vi "Excel_Voltage.vi"(7 "duanVoltage":dbl[](array[numeric]), 8 "error in (no error)":errorcluster, 10 "Report path in":path, 11 "report in":refnum<class "NI_report.lvclass">) -> (0 "error out":errorcluster, 2 "Report path out":path, 3 "report out":refnum<class "NI_report.lvclass">)   [LabVIEW 2015]
doc: "如果duanVoltage=-1，报表中输出‘-’。"
uses:
  <vilib>/Utility/NIReport.llb/NI_report.lvclass
  <vilib>/addons/_office/NI_ReportGenerationToolkit.lvlib
panel:
  in  "start(-1,-1)":cluster{"row":i32, "column":i32}
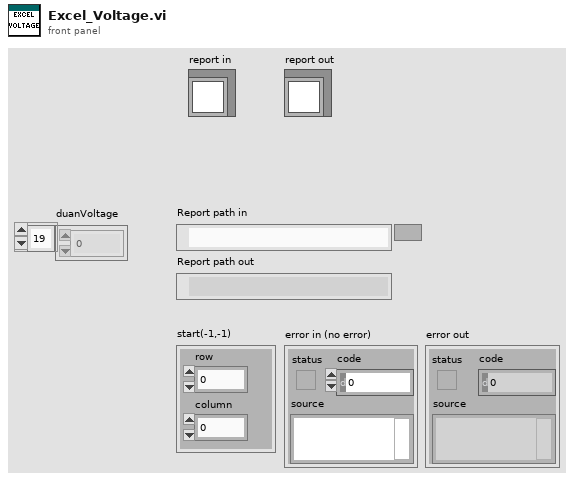
[diagram p1: front panel]
types:
  T1 = enum16{"Standard Report", "HTML", "Word", "Excel"}
  T2 = enum16{"maximized", "minimized", "normal", "no change"}
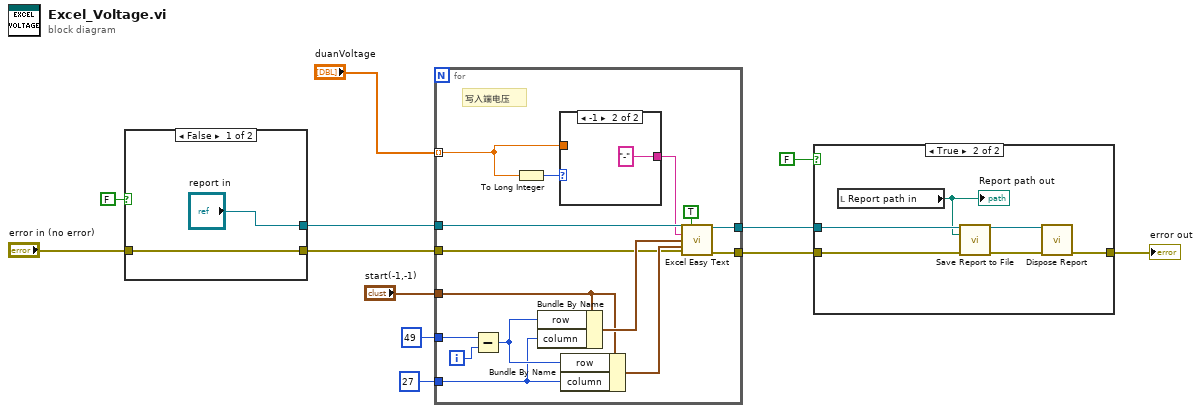
[diagram p0: block diagram]
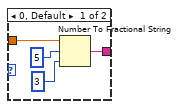
[diagram p2: hidden frame]
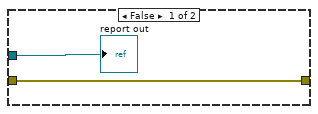
[diagram p3: hidden frame]
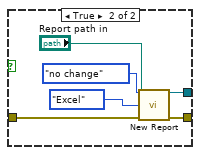
[diagram p4: hidden frame]
diagram:
  n1 = case shown="False" FALSE {
    tunnel: ["report in" w17] -> w12
    tunnel: [w14 w16] -> w11
    tunnel: "error in (no error)" -> [w14 w15]
    frame False {
    }
    frame True {
      n2 = call <vilib>:"New Report.vi"("window state (normal)"=T2."no change", "report type"=T1."Excel", "template (empty)"="Report path in", "error in (no error)"=w15) -> ("report out"=w17:refnum<class "NI_report.lvclass">, "error out"=w16:errorcluster)  [unwired: 10 in]
    }
  }
  n3 = for {
    tunnel: w12 -> [w31]
    tunnel: w11 -> [w30]
    tunnel: [w29] -> w10
    tunnel: [w28] -> w9
    tunnel: "start(-1,-1)" -> [w26]
    tunnel: 49 ("row") -> [w25]
    tunnel: 27 ("column") -> [w24]
    tunnel: "duanVoltage" -> [w23] mode=indexing
    i -> [w33]
    # "写入端电压"
    n4 = Subtract(x=w25, y=w33) -> (x-y=w32:i32)
    n5 = To Long Integer(number=w23) -> (32bit integer=w21:i32)
    n6 = Bundle By Name(cluster=w26, "row"=w32, "column"=w24) -> (w35:cluster{"row":i32, "column":i32})
    n7 = case shown="-1" w21 {
      tunnel: [w39 "-"] -> w27
      tunnel: w23 -> [w36 _]
      frame 0, Default {
        n8 = Number To Fractional String(number=w36, width (-)=i16 5, precision (6)=i16 3 ("width (-)")) -> (F-format string=w39:string)  [unwired: 1 in]
      }
      frame -1 {
      }
    }
    n9 = Bundle By Name(cluster=w26, "row"=w32, "column"=w24) -> (w34:cluster{"row":i32, "column":i32})
    n10 = call <vilib>:"Excel Easy Text.vi"("report in"=w31, "border? (F)"=TRUE, "text"=w27, "start (-1, -1)"=w35, "end (-1, -1)"=w34, "error in (no error)"=w30) -> ("report out"=w29:refnum<class "NI_report.lvclass">, "error out"=w28:errorcluster)  [unwired: 5 in, 3 out]
  }
  n11 = case shown="True" FALSE {
    tunnel: w10 -> [w41 w46]
    tunnel: w9 -> [w42 w45]
    tunnel: [w42 w44] -> w7
    frame False {
      "report out" <- w41
    }
    frame True {
      n12 = local read "Report path in"() -> (w43:path)
      "Report path out" <- w43
      n13 = call-dynamic "Save Report to File.vi"("report in"=w46, "report file path"=w43, "error in (no error)"=w45) -> ("report out"=w48:refnum<class "NI_report.lvclass">, "error out"=w47:errorcluster)  [unwired: 11 in]
      n14 = call-dynamic "Dispose Report.vi"("report in"=w48, "error in (no error)"=w47) -> ("error out"=w44:errorcluster)  [unwired: 13 in]
    }
  }
  "error out" <- w7
